vi "Aync Colored.vi"() -> ()   [LabVIEW 2018]
panel:
  out "Fibonacci(n)":u32
  in  "n":u32
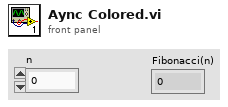
[diagram p1: front panel]
types:
  T1 = typedef "imagedata.ctl" = cluster{"image type":i32, "image depth":i32, "image":u8[], "mask":u8[], "colors":u32[], "Rectangle":cluster{"left":i16, "top":i16, "right":i16, "bottom":i16}}
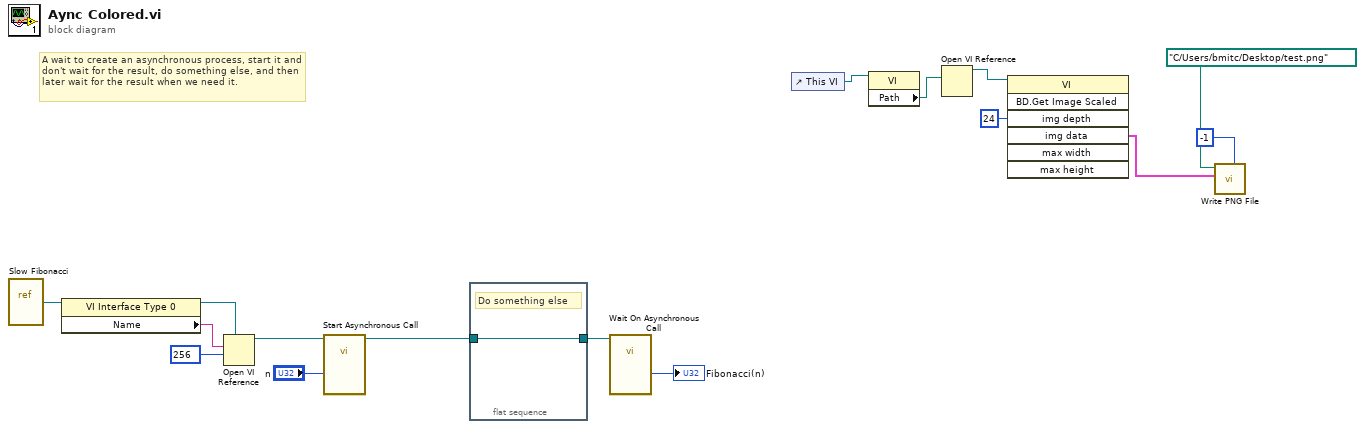
[diagram p0: block diagram]
diagram:
  # "A wait to create an asynchronous process, start it and don't wait for the result, do something else, and then later wait for the result when we need it."
  # "-"
  # "-"
  n1 = vi-ref "Slow Fibonacci.vi"() -> (w11:refnum<vi>)
  n2 = property class="VI Interface Type 0"(reference=w11) -> (reference out=w12:refnum<vi>, "Name"=w13:string)  [unwired: 1 in, 1 out]
  n3 = Open VI Reference(type specifier VI Refnum (for type only)=w12, vi path=w13, options=256) -> (vi reference=w10:refnum<vi>)  [unwired: 3 in, 1 out]
  n4 = call-by-ref "Start Asynchronous Call"(reference=w10, "n"="n") -> (reference out=w9:refnum<vi>)  [unwired: 1 in, 2 out]
  n5 = flat-sequence {
    tunnel: w9 -> [w17]
    tunnel: [w17] -> w8
    frame #0 {
      # "Do something else"
    }
  }
  n6 = call-by-ref "Wait On Asynchronous Call"(reference=w8) -> ("Fibonacci(n)"=→"Fibonacci(n)":u32)  [unwired: 2 in, 2 out]
  n7 = control-ref of="This VI"() -> (w7:refnum<vi>)
  n8 = property class="VI"(reference=w7) -> ("Path"=w6:path)  [unwired: 1 in, 2 out]
  n9 = Open VI Reference(vi path=w6) -> (vi reference=w5:refnum<vi>)  [unwired: 5 in, 1 out]
  n10 = invoke class="VI" method="BD.Get Image Scaled"(reference=w5, "img depth"=24 ("Image Depth")) -> ("img data"=w3:T1)  [unwired: 5 in, 6 out]
  n11 = call <vilib>:"Write PNG File.vi"("compression (default)"=-1, "image data"=w3, "path to PNG file"=path "C:/Users/bmitc/Desktop/test.png") -> ()  [unwired: 7 in, 2 out]
